vi "thold_clamp.vi"() -> ()   [LabVIEW 2017]
panel:
  out "Distance (calibrated) (Clamp (Rake) 2)":sgl format="%.2f"
  out "Edge Coordinates (calibrated) (Clamp (Rake) 2)":cluster{"X":sgl, "Y":sgl}[](array[cluster]) {"Y" format="%.2f"; "X" format="%.2f"}
  out "Distance (calibrated) (Clamp (Rake) 1)":sgl format="%.2f"
  out "Edge Coordinates (calibrated) (Clamp (Rake) 1)":cluster{"X":sgl, "Y":sgl}[](array[cluster]) {"Y" format="%.2f"; "X" format="%.2f"}
  out "Distance (Clamp (Rake) 2)":sgl format="%.2f"
  out "Edge Coordinates (Clamp (Rake) 2)":cluster{"X":sgl, "Y":sgl}[](array[cluster]) {"Y" format="%.2f"; "X" format="%.2f"}
  out "Distance (Clamp (Rake) 1)":sgl format="%.2f"
  out "Edge Coordinates (Clamp (Rake) 1)":cluster{"X":sgl, "Y":sgl}[](array[cluster]) {"Y" format="%.2f"; "X" format="%.2f"}
  in  "Stop (F)":bool
  out "Image Out":T1(plugin-control)
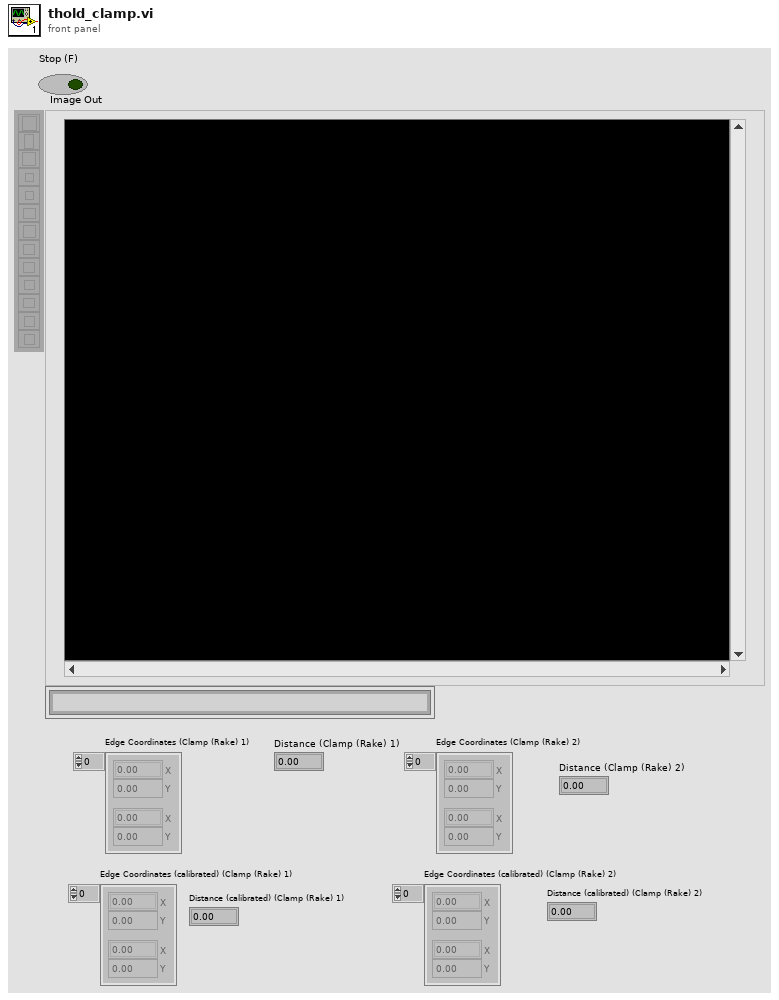
[diagram p1: front panel]
types:
  T1 = typedef "IMAQ Image.ctl" = refnum<image>
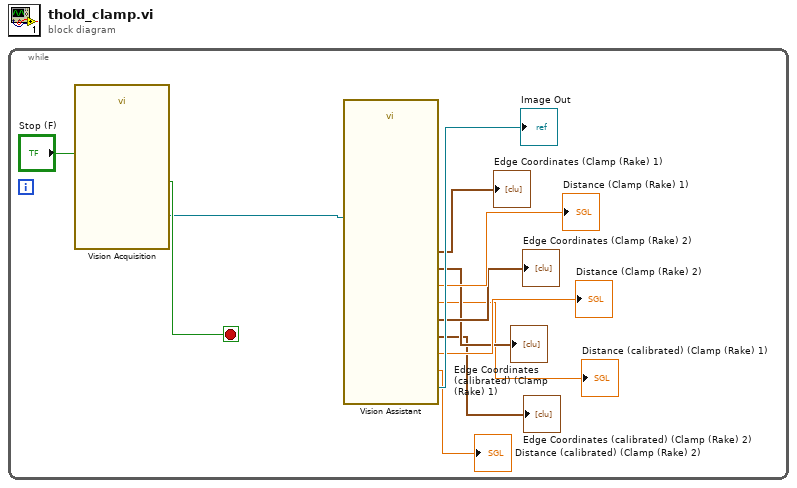
[diagram p0: block diagram]
diagram:
  n1 = while {
    stop <- w11 stop-if-true
    n2 = call "Vision Acquisition"("Stop (F)"="Stop (F)") -> ("Image Out"=w1:T1, "Stopped"=w11:bool)  [unwired: 24 in, 1 out]
    n3 = call "Vision Assistant"("Image In"=w1) -> ("Distance (calibrated) (Clamp (Rake) 2)"=→"Distance (calibrated) (Clamp (Rake) 2)":sgl, "Edge Coordinates (calibrated) (Clamp (Rake) 2)"=→"Edge Coordinates (calibrated) (Clamp (Rake) 2)":cluster{"X":sgl, "Y":sgl}[], "Image Out"=→"Image Out":T1, "Edge Coordinates (Clamp (Rake) 1)"=→"Edge Coordinates (Clamp (Rake) 1)":cluster{"X":sgl, "Y":sgl}[], "Distance (Clamp (Rake) 1)"=→"Distance (Clamp (Rake) 1)":sgl, "Edge Coordinates (Clamp (Rake) 2)"=→"Edge Coordinates (Clamp (Rake) 2)":cluster{"X":sgl, "Y":sgl}[], "Distance (Clamp (Rake) 2)"=→"Distance (Clamp (Rake) 2)":sgl, "Edge Coordinates (calibrated) (Clamp (Rake) 1)"=→"Edge Coordinates (calibrated) (Clamp (Rake) 1)":cluster{"X":sgl, "Y":sgl}[], "Distance (calibrated) (Clamp (Rake) 1)"=→"Distance (calibrated) (Clamp (Rake) 1)":sgl)  [unwired: 17 in, 1 out]
  }
